vi "Process.vi"(8 "error in":errorcluster, 11 "SMO.Example":refnum<class "SMO.TopLevel.lvclass">) -> (0 "error out":errorcluster, 3 "SMO.Example out":refnum<class "SMO.TopLevel.lvclass">)   [LabVIEW 2013, in "SMO.TopLevel.lvclass"]
doc: "---------------------------------------------------------------\nJKI State Machine Objects™\nhttp://jki.net/state-machine-objects/\nCopyright (C) 2005-2015, JKI <info@jki.net>\nALL RIGHTS RESERVED"
uses:
  SMO.TopLevel.lvclass
  src/SMO/Typedefs/Parent Call--Enum.ctl
  src/SMO/SMO.lvclass
panel:
  # "For instructions on how to use the JKI State Machine Objects, examples and video tutorials, visit:\nhttp://jki.net/state-machine-objects/\n\nJKI State Machine Objects™\nhttp://jki.net/state-machine-objects/\nCopyright (C) 2005-2015, JKI <info@jki.net>\nALL RIGHTS RESERVED"
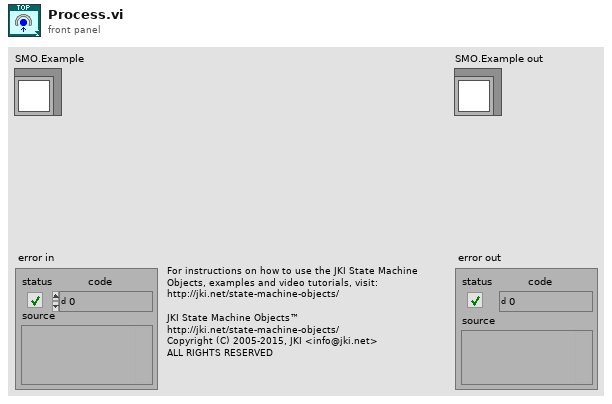
[diagram p1: front panel]
types:
  T1 = typedef "SMO.lvclass/Parent Call--Enum.ctl" = enum16{"Allows parent to run", "Does not request parent to run"}
  T2 = enum32{"invalid app kind", "Development System", "Run Time System", "Student Edition", "Embedded LabVIEW", "Evaluation", "Custom"}
  T3 = enum32{"Invalid", "Standard", "Closed", "Hidden", "Minimized", "Maximized"}
  T4 = cluster{"Core":cluster{"Current VI Reference":refnum<vi>, "Close Panel on Exit?":bool, "error":errorcluster}, "Self Ref":refnum<class "SMO.TopLevel.lvclass">, "Your string data":string, "Pump State":bool, "Valve 1 State":bool, "Flow 1 Actual":dbl, "Flow 2 Actual":dbl, "Flow 1 Target":dbl, "Flow 2 Target":dbl}
  T5 = cluster{"Current VI Reference":refnum<vi>, "Close Panel on Exit?":bool, "error":errorcluster}
  T6 = typedef "SMO.lvclass/Protected Events.ctl" = cluster{"StopProcesses":refnum<user-event>, "AbortProcesses":refnum<user-event>, "Config Changed":refnum<user-event>}
  T7 = typedef "SMO.TopLevel.lvclass/ProtectedEvents--Cluster.ctl" = cluster{"API_Template":refnum<user-event>, "PumpState":refnum<user-event>, "Valve State":refnum<user-event>}
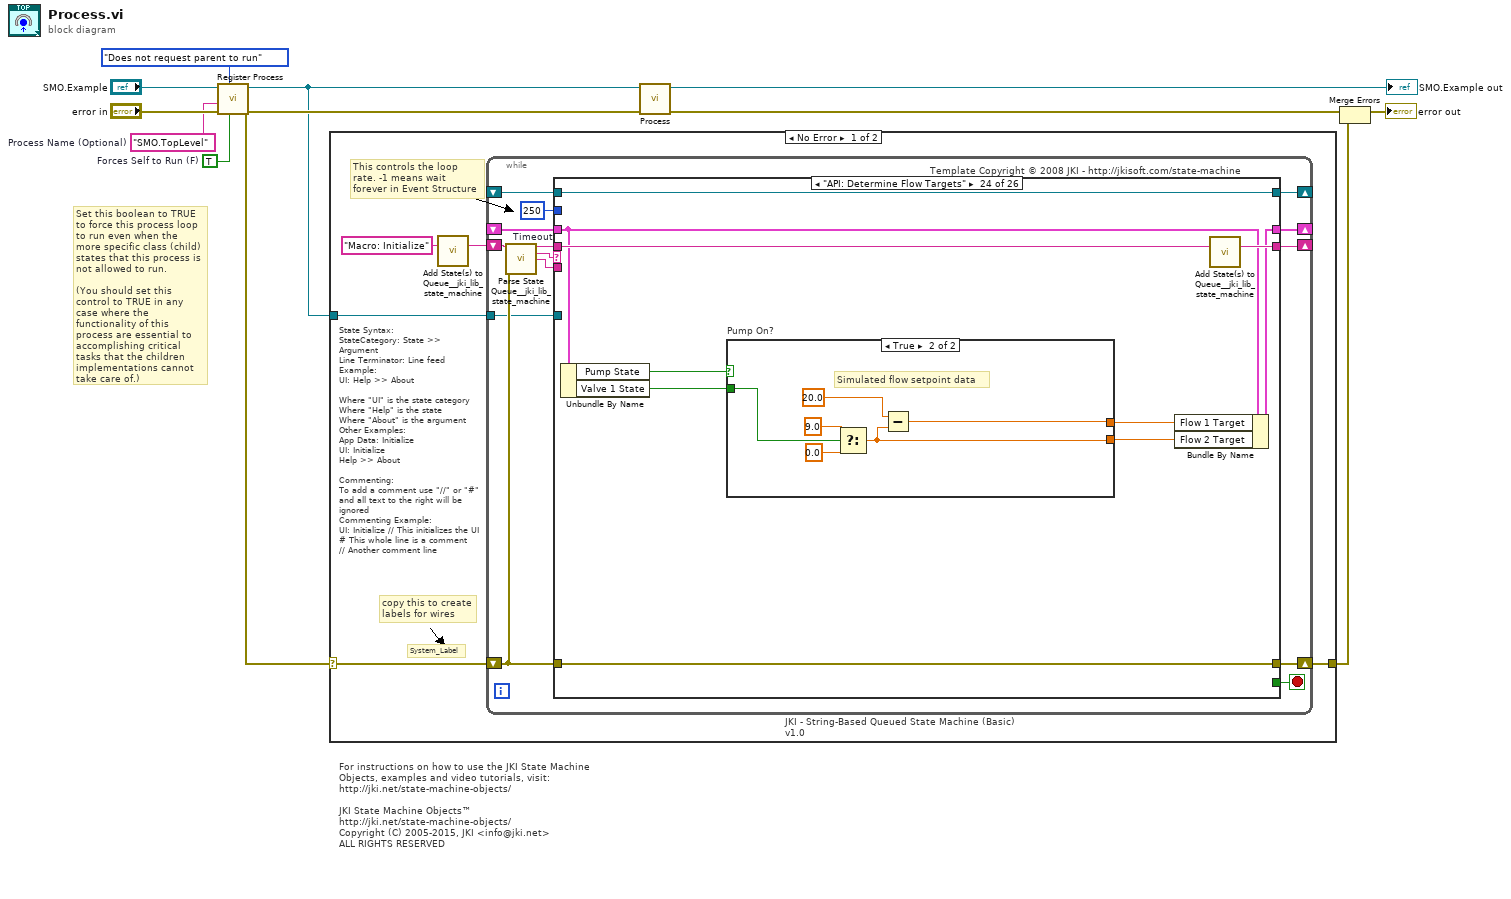
[diagram p0: block diagram]
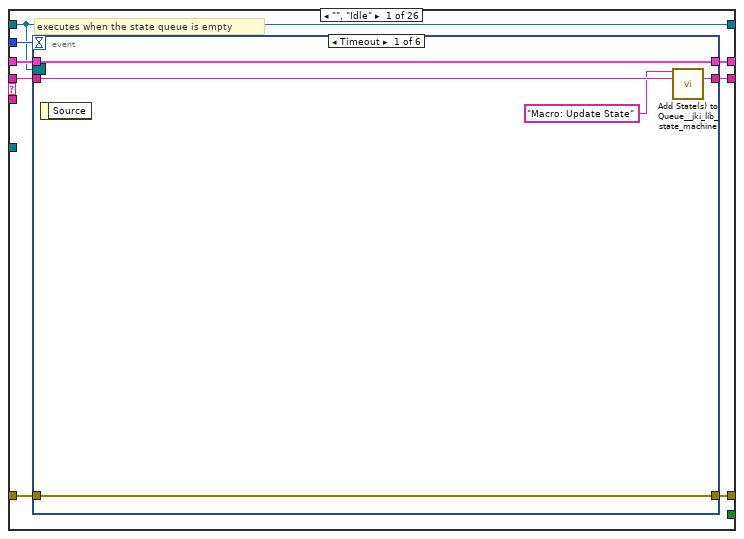
[diagram p2: hidden frame]
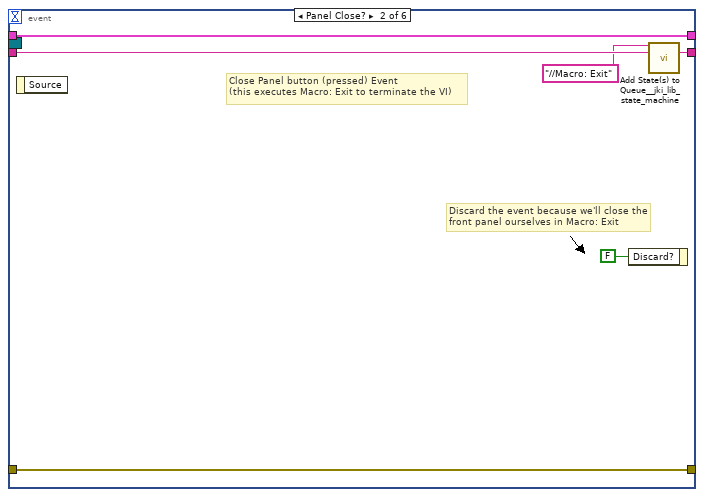
[diagram p3: hidden frame]
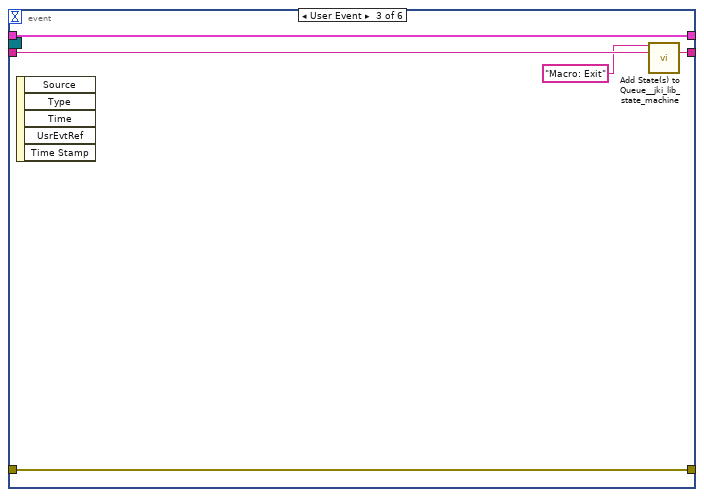
[diagram p4: hidden frame]
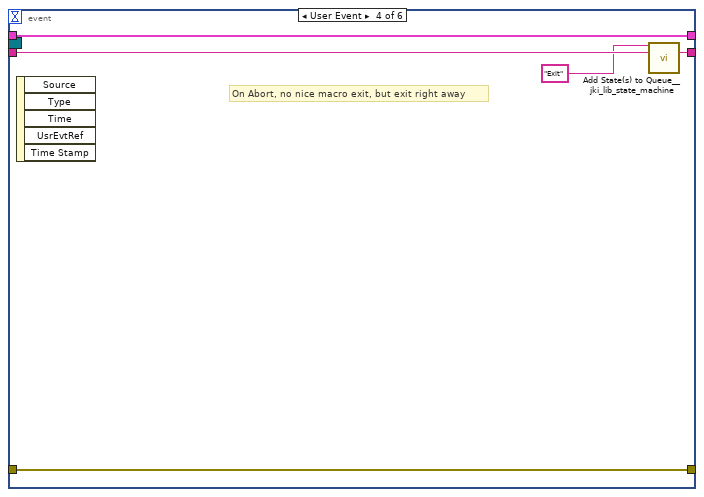
[diagram p5: hidden frame]
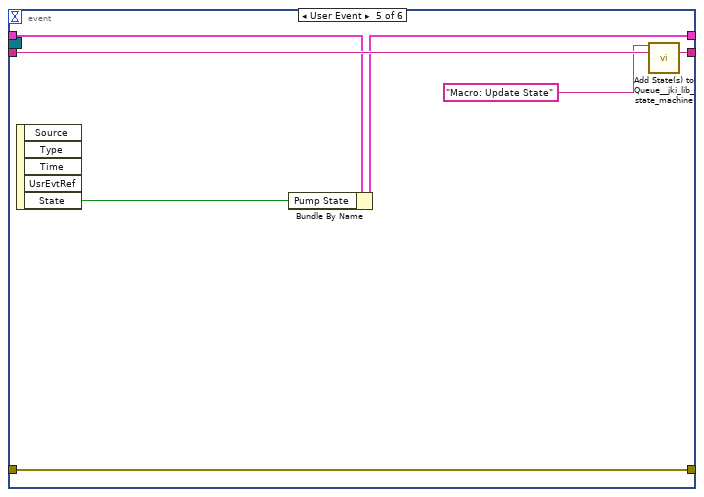
[diagram p6: hidden frame]
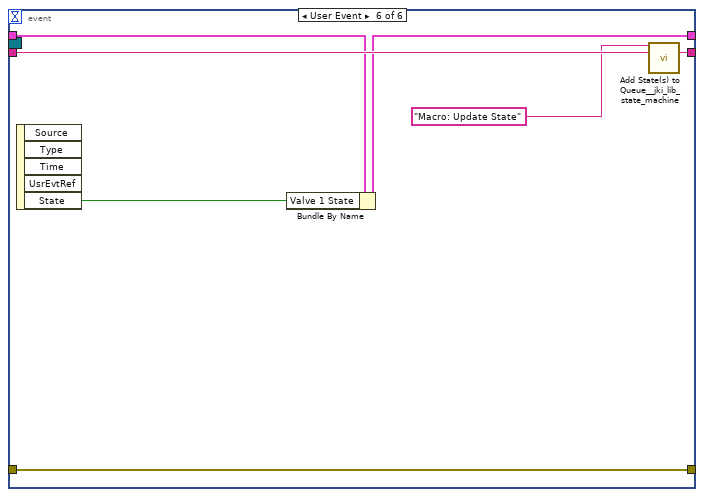
[diagram p7: hidden frame]
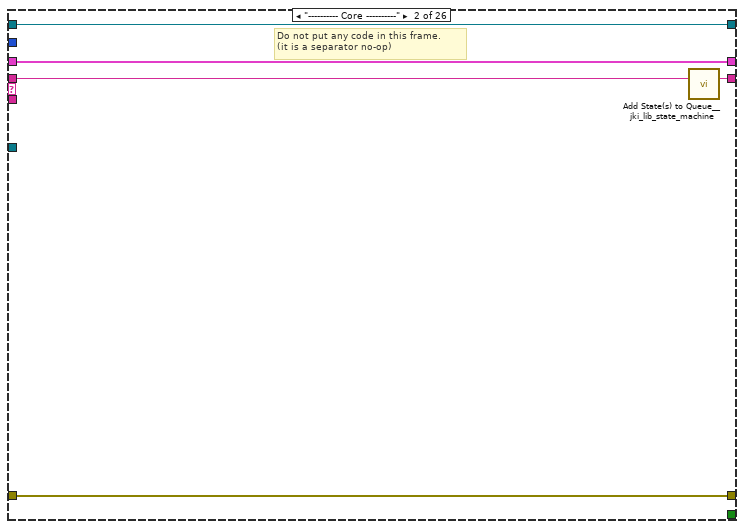
[diagram p8: hidden frame]
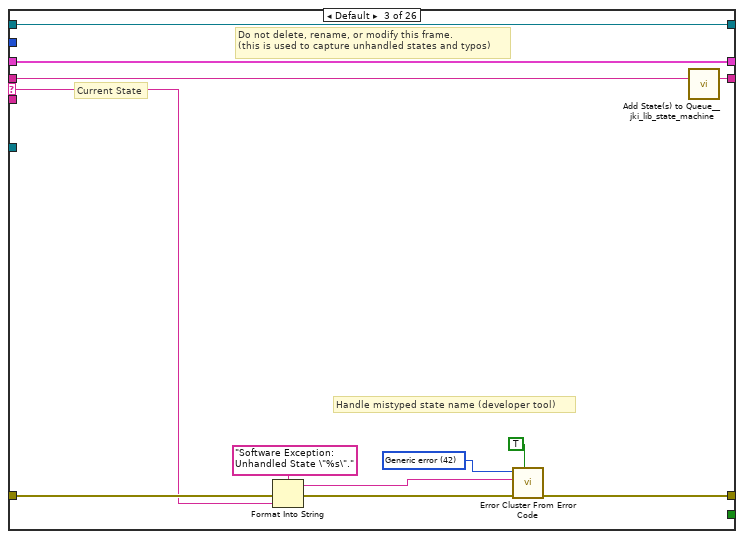
[diagram p9: hidden frame]
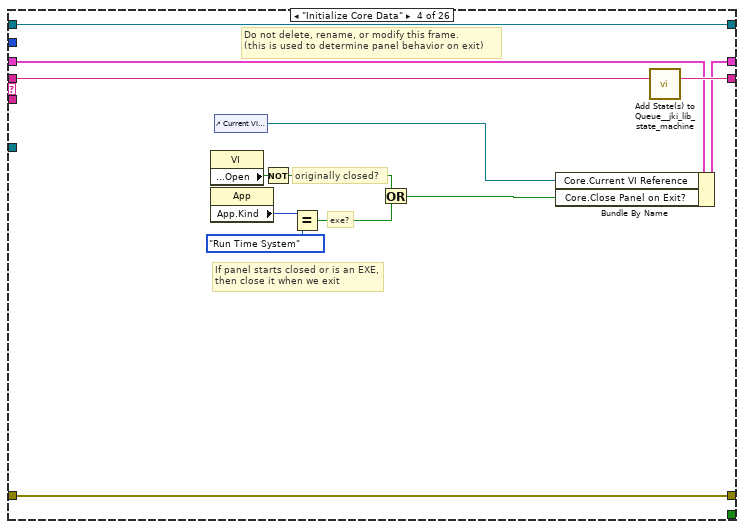
[diagram p10: hidden frame]
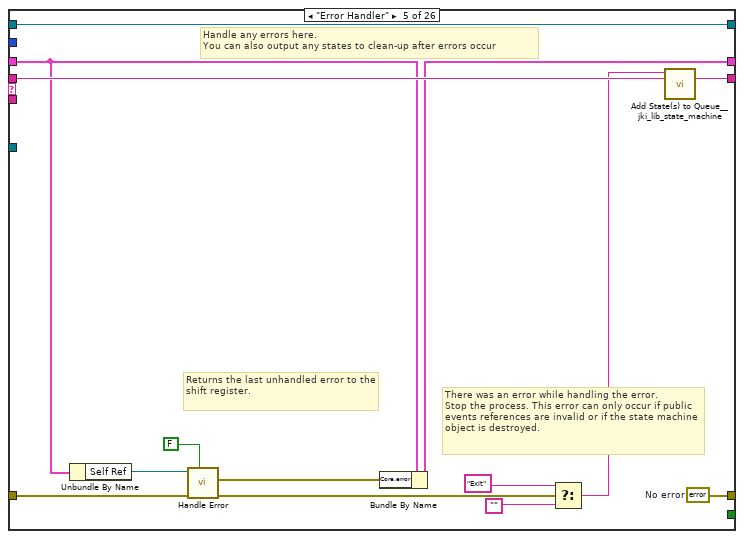
[diagram p11: hidden frame]
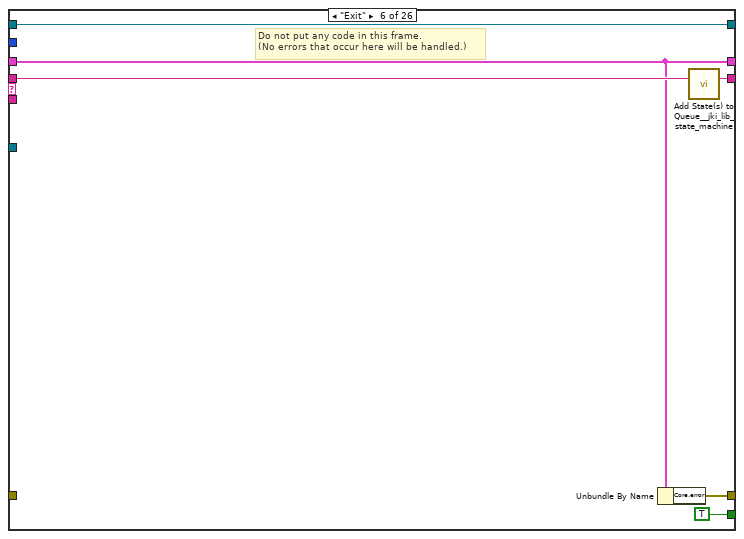
[diagram p12: hidden frame]
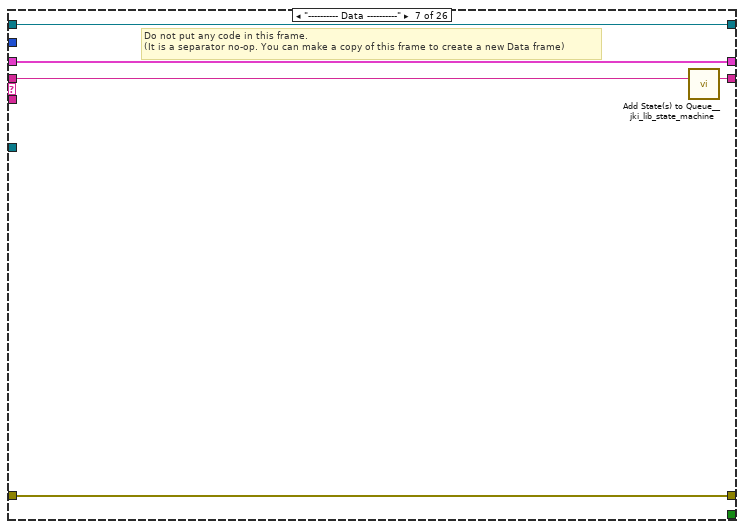
[diagram p13: hidden frame]
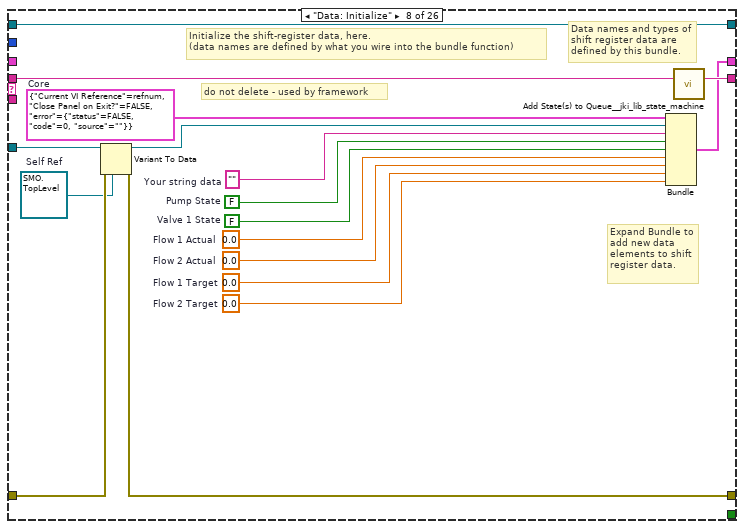
[diagram p14: hidden frame]
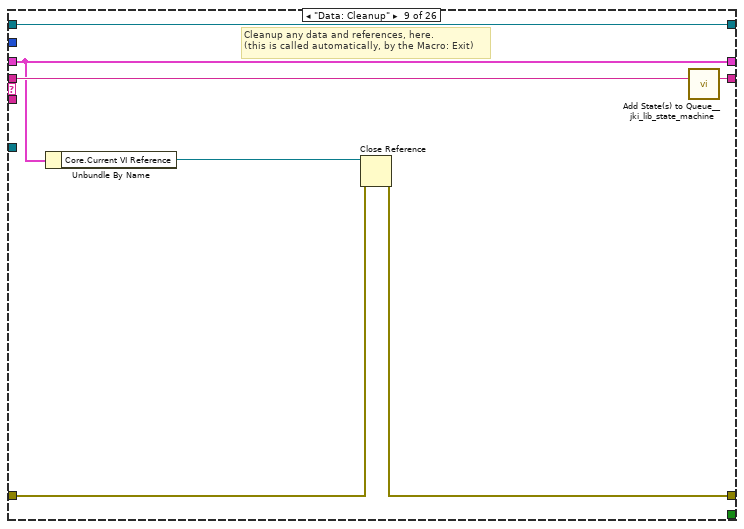
[diagram p15: hidden frame]
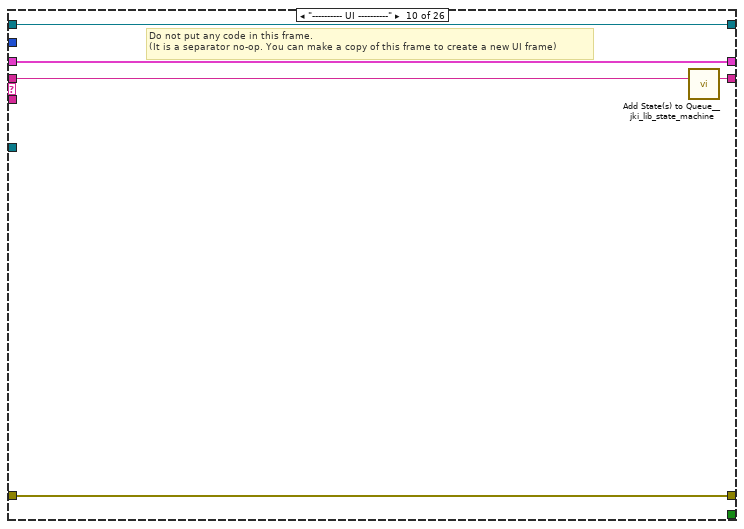
[diagram p16: hidden frame]
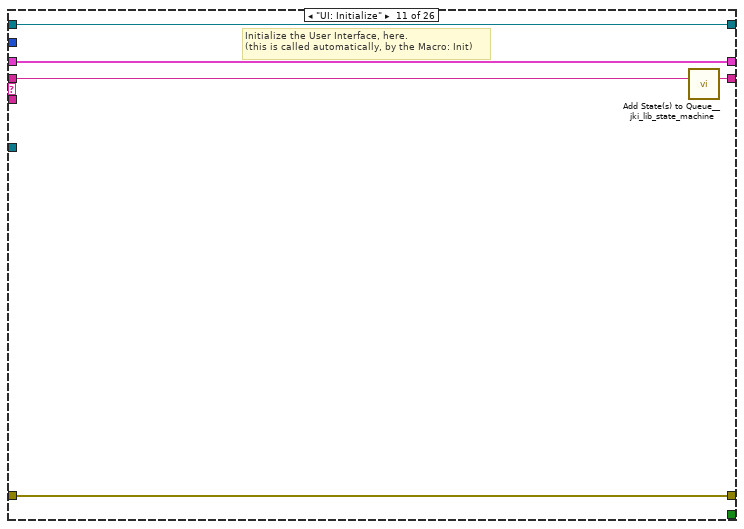
[diagram p17: hidden frame]
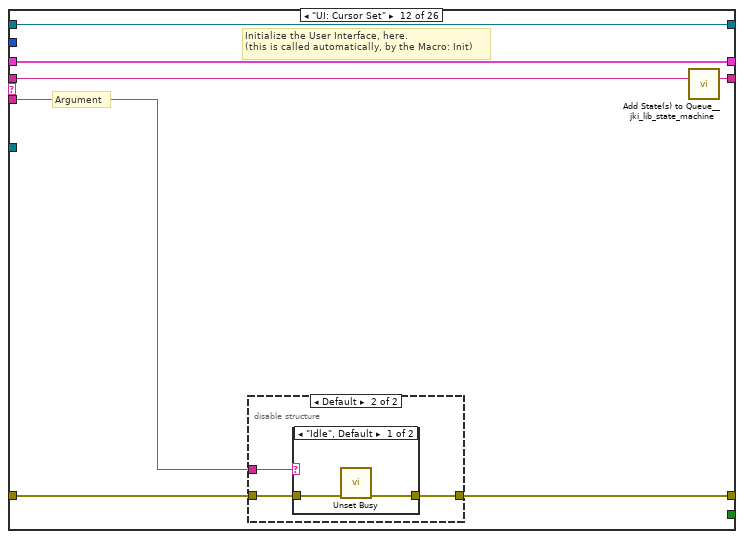
[diagram p18: hidden frame]
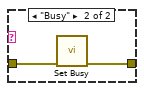
[diagram p20: hidden frame]
diagram:
  w1 = TRUE  # Forces Self to Run (F)
  w2 = "SMO.TopLevel"  # Process Name (Optional)
  # "Set this boolean to TRUE to force this process loop to run even when the more specific class (child) states that this process is not allowed to run.\n\n(You should set this control to TRUE in any case where the functionality of this process are essential to accomplishing critical tasks that the children implementations cannot take care of.)"
  # "For instructions on how to use the JKI State Machine Objects, examples and video tutorials, visit:\nhttp://jki.net/state-machine-objects/\n\nJKI State Machine Objects™\nhttp://jki.net/state-machine-objects/\nCopyright (C) 2005-2015, JKI <info@jki.net>\nALL RIGHTS RESERVED"
  n1 = call "Register Process.vi"("Forces Self to Run (F)"=w1, "Parent Call"=Parent_Call--Enum."Does not request parent to run", "error in (no error)"="error in", "Process Name (optional)"=w2, "SMO"="SMO.Example") -> ("error out"=w8:errorcluster, "SMO out"=w7:refnum<class "SMO.TopLevel.lvclass">)  [unwired: 5 in]
  n2 = case shown="No Error" w8 {
    selector: w8 -> [w13 w347]
    tunnel: w7 -> [w14 _]
    tunnel: [w12 w347] -> w4
    frame No Error {
      # "State Syntax:\nStateCategory: State >> Argument\nLine Terminator: Line feed\nExample:\nUI: Help >> About\n\nWhere \"UI\" is the state category\nWhere \"Help\" is the state\nWhere \"About\" is the argument\nOther Examples:\nApp Data: Initialize\nUI: Initialize\nHelp >> About\n\nCommenting:\nTo add a comment use \"//\" or \"#\" and all text to the right will be ignored\nCommenting Example:\nUI: Initialize // This initializes the UI\n# This whole line is a comment\n// Another comment line"
      # "copy this to create labels for wires"
      # "This controls the loop rate. -1 means wait forever in Event Structure"
      # "System_Label"
      n3 = call <vilib>:"Add State(s) to Queue__jki_lib_state_machine.vi"("State(s) in (\"\")"="Macro: Initialize") -> ("States Out"=w16:string)  [unwired: 14 in]
      n4 = while "JKI - String-Based Queued State Machine (Basic) v1.0" {
        shift-right: [w23] -> _
        shift-left: _ -> [w22]
        shift-right: [w26] -> w12
        shift-left: w13 -> [w20]
        shift-right: [w25] -> _
        shift-left: w16 -> [w27]
        tunnel: w14 -> [w19]
        shift-right: [w18] -> _
        shift-left: _ -> [w17]
        stop <- w24 stop-if-true
        w21 = 250  # Timeout
        # "Template Copyright © 2008 JKI - http://jkisoft.com/state-machine"
        n5 = call <vilib>:"Parse State Queue__jki_lib_state_machine.vi"("State Queue"=w27, "Error In (no error)"=w20) -> ("Remaining States"=w29:string, "Current State"=w30:string, "Arguments"=w28:string)  [unwired: 11 in]
        n6 = case shown="\"API: Determine Flow Targets\"" w30 {
          selector: w30 -> [_ _ w80 _ _ _ _ _ _ _ _ _ _ _ _ _ _ _ _ _ _ _ _ _ _ _]
          tunnel: w29 -> [w38 w78 w84 w103 w117 w123 w128 w145 w152 w157 w162 w169 w185 w217 w223 w232 w246 w251 w262 w267 w280 w286 w291 w301 w337 w346]
          tunnel: w28 -> [_ _ _ _ _ _ _ _ _ _ _ w163 w178 _ _ _ _ _ _ _ _ _ _ _ _ _]
          tunnel: w22 -> [w36 w75 w82 w94 w108 w119 w125 _ w147 w154 w160 w167 w183 w214 w220 w228 w237 w248 w259 w264 w278 w284 w289 w295 w333 w343]
          tunnel: [w35 w76 w86 w100 w105 w118 w126 w140 w148 w155 w159 w164 w179 w215 w221 w230 w244 w249 w253 w265 w268 w282 w287 w296 w334 w340] -> w26
          tunnel: w20 -> [w34 w76 w85 w100 w109 _ w126 w141 w149 w155 w159 w165 w180 w215 w221 w230 w244 w249 w254 w265 w269 w282 w287 w296 w334 w341]
          tunnel: [w37 w77 w83 w102 w116 w122 w127 w144 w151 w156 w161 w168 w184 w216 w222 w231 w245 w250 w261 w266 w279 w285 w290 w300 w336 w345] -> w25
          tunnel: [_ _ _ _ _ TRUE _ _ _ _ _ _ _ _ _ _ _ _ _ _ _ _ _ _ _ _] -> w24
          tunnel: [w33 w75 w82 w101 w107 w119 w125 w143 w147 w154 w160 w167 w183 w214 w220 w228 w237 w248 w259 w264 w278 w284 w289 w294 w332 w343] -> w23
          tunnel: w21 -> [w32 _ _ _ _ _ _ _ _ _ _ _ _ _ _ _ _ _ _ _ _ _ _ _ _ _]
          tunnel: w19 -> [_ _ _ _ _ _ _ w138 _ _ _ _ _ _ _ _ _ _ _ _ _ _ _ _ _ _]
          tunnel: [w31 w74 w79 w91 w115 w120 w124 w136 w146 w153 w158 w166 w182 w213 w219 w229 w238 w247 w260 w263 w274 w283 w288 w299 w335 w344] -> w18
          tunnel: w17 -> [w31 w74 w79 w91 w115 w120 w124 w136 w146 w153 w158 w166 w182 w213 w219 w229 w238 w247 w260 w263 _ w283 w288 w299 w335 w344]
          frame "", "Idle" {
            # "executes when the state queue is empty"
            n7 = event shown="[0] Timeout" {
              selector: w31 -> [_ _ _ _ _ _]
              dyn-events: _ -> [_ _ _ _ _ _]
              timeout: w32 -> [_ _ _ _ _ _]
              tunnel: w38 -> [w43 w49 w54 w59 w66 w73]
              tunnel: [w42 w48 w53 w58 w65 w72] -> w37
              tunnel: w36 -> [w40 w46 w51 w56 w63 w70]
              tunnel: [w41 w47 w52 w57 w64 w71] -> w35
              tunnel: w34 -> [w41 w47 w52 w57 w64 w71]
              tunnel: [w40 w46 w51 w56 w62 w69] -> w33
              event Timeout {
                n8 = event-data() -> ()  [unwired: 1 in, 1 out]
                n9 = call <vilib>:"Add State(s) to Queue__jki_lib_state_machine.vi"("State(s) in Front (\"\")"="Macro: Update State", "State(s) in (\"\")"=w43) -> ("States Out"=w42:string)  [unwired: 13 in]
              }
              event Panel Close? {
                # "Discard the event because we'll close the front panel ourselves in Macro: Exit"
                # "Close Panel button (pressed) Event\n(this executes Macro: Exit to terminate the VI)"
                n10 = event-data() -> ()  [unwired: 1 in, 1 out]
                n11 = event-data("Discard?"=FALSE) -> ()  [unwired: 1 in, 1 out]
                n12 = call <vilib>:"Add State(s) to Queue__jki_lib_state_machine.vi"("State(s) in Front (\"\")"="//Macro: Exit", "State(s) in (\"\")"=w49) -> ("States Out"=w48:string)  [unwired: 13 in]
              }
              event User Event {
                n13 = event-data() -> ()  [unwired: 1 in, 5 out]
                n14 = call <vilib>:"Add State(s) to Queue__jki_lib_state_machine.vi"("State(s) in Front (\"\")"="Macro: Exit", "State(s) in (\"\")"=w54) -> ("States Out"=w53:string)  [unwired: 13 in]
              }
              event User Event {
                # "On Abort, no nice macro exit, but exit right away"
                n15 = event-data() -> ()  [unwired: 1 in, 5 out]
                n16 = call <vilib>:"Add State(s) to Queue__jki_lib_state_machine.vi"("State(s) in Front (\"\")"="Exit", "State(s) in (\"\")"=w59) -> ("States Out"=w58:string)  [unwired: 13 in]
              }
              event User Event {
                n17 = event-data() -> ("State"=w60:bool)  [unwired: 1 in, 4 out]
                n18 = Bundle By Name(cluster=w63, "Pump State"=w60) -> (w62:T4)
                n19 = call <vilib>:"Add State(s) to Queue__jki_lib_state_machine.vi"("State(s) in Front (\"\")"="Macro: Update State", "State(s) in (\"\")"=w66) -> ("States Out"=w65:string)  [unwired: 13 in]
              }
              event User Event {
                n20 = event-data() -> ("State"=w67:bool)  [unwired: 1 in, 4 out]
                n21 = Bundle By Name(cluster=w70, "Valve 1 State"=w67) -> (w69:T4)
                n22 = call <vilib>:"Add State(s) to Queue__jki_lib_state_machine.vi"("State(s) in Front (\"\")"="Macro: Update State", "State(s) in (\"\")"=w73) -> ("States Out"=w72:string)  [unwired: 13 in]
              }
            }
          }
          frame "---------- Core ----------" {
            # "Do not put any code in this frame.\n(it is a separator no-op)"
            n23 = call <vilib>:"Add State(s) to Queue__jki_lib_state_machine.vi"("State(s) in (\"\")"=w78) -> ("States Out"=w77:string)  [unwired: 14 in]
          }
          frame Default {
            w89 = 42 items=["No error", "Argument error", "Memory is full", "Out of zone", "End of file", "File already open", "Generic file I/O error", "File not found", "File permission error", "Disk is full", "Duplicate path", "Too many files open", "System feature not enabled", "Resource file not found", "Cannot add resource", "Resource not found", "Image not found", "Image memory error", "Pen does not exist", "Config type invalid", "Config token not found", "Config parse error", "Config memory error", "Bad external code format", "Bad external code offset", "External code not present", "Null window", "Destroy window error", "Null menu", "Print aborted", "Bad print record", "Print driver error", "Windows error during printing", "Memory error during printing", "Print dialog error", "Generic print error", "Invalid device refnum", "Device not found", "Device parameter error", "Device unit error", "Cannot open device", "Device call aborted", "Generic error", "Cancelled by user", "Object ID too low", "Object ID too high", "Object not in heap", "Unknown heap", "Unknown object (invalid DefProc)", "Unknown object (DefProc not in table)", "Message out of range", "Invalid (null) method", "Unknown message", "Manager call not supported", "Bad address", "Network operation in progress", "Network operation timed out", "Connection is busy", "Network attribute not supported", "Network error", "Address in use", "System out of memory", "Connection aborted", "Connection refused", "Not connected", "Already connected", "Connection closed", "Initialization error (interapplication manager)", "Bad occurrence", "Wait on unbound occurrence handler", "Occurrence queue overflow", "Datalog type conflict", "Unused", "Unrecognized type (interapplication manager)", "Memory corrupt", "Failed to make temporary DLL", "Old CIN version", "Drag socket not found", "Failed to load drop-object", "Failed to register OLE object", "Failed to release OLE object", "Format specifier type mismatch", "Unknown format specifier", "Too few format specifiers", "Too many format specifiers", "Scan failed", "Newer CIN version", "Error converting to variant", "Runtime menu error", "Password tampered", "Variant attribute not found", "Incompatible variant data type", "Event data is not available", "Event Store is not present", "Occurrence is not found", "Event Queue is not created", "Event info is not available", "Refnum passed is NULL", "Error retrieving Class GUID", "Error retrieving CoClass GUID", "Error retrieving TypeLib GUID.", "Bad built application magic bytes.", "Specific driver is different from the specific driver associated with the Logical Name.", "There is no session opened to the class driver.", "Max Error", "MAX - Error with config objects", "MAX - Error loading configuration", "MAX - Group not supported"]
            # "Current State"
            # "Do not delete, rename, or modify this frame.\n(this is used to capture unhandled states and typos)"
            # "Handle mistyped state name (developer tool)"
            n24 = Format Into String(format string="Software Exception: Unhandled State \"%s\"." ("message"), error in=w85, w80) -> (resulting string=w88:string, error out=w87:errorcluster)  [unwired: 1 in]
            n25 = call <vilib>:"Error Cluster From Error Code.vi"("show call chain? (False)"=TRUE, "error in (no error)"=w87, "error message (\"\")"=w88, "error code (0)"=w89) -> ("error out"=w86:errorcluster)  [unwired: 5 in]
            n26 = call <vilib>:"Add State(s) to Queue__jki_lib_state_machine.vi"("State(s) in (\"\")"=w84) -> ("States Out"=w83:string)  [unwired: 14 in]
          }
          frame "Initialize Core Data" {
            # "Do not delete, rename, or modify this frame.\n(this is used to determine panel behavior on exit)"
            # "originally closed?"
            # "exe?"
            # "If panel starts closed or is an EXE, then close it when we exit"
            n27 = property class="VI"() -> ("Front Panel.Open"=w99:bool)  [unwired: 2 in, 2 out]
            n28 = property class="App"() -> ("App.Kind"=w98:T2)  [unwired: 2 in, 2 out]
            n29 = control-ref of="Current VI Reference"() -> (w92:refnum<vi>)
            n30 = Not(x=w99) -> (.not. x?=w96:bool)
            n31 = Equal?(x=w98, y=T2."Run Time System" ("Application:Kind")) -> (x = y?=w95:bool)
            n32 = Or(x=w96, y=w95) -> (x .or. y?=w93:bool)
            n33 = Bundle By Name(cluster=w94, "Core.Current VI Reference"=w92, "Core.Close Panel on Exit?"=w93) -> (w101:T4)
            n34 = call <vilib>:"Add State(s) to Queue__jki_lib_state_machine.vi"("State(s) in (\"\")"=w103) -> ("States Out"=w102:string)  [unwired: 14 in]
          }
          frame "Error Handler" {
            w105 = errorcluster {"status"=FALSE, "code"=0, "source"=""}  # No error
            # "Returns the last unhandled error to the shift register."
            # "There was an error while handling the error.\nStop the process. This error can only occur if public events references are invalid or if the state machine object is destroyed."
            # "Handle any errors here.\nYou can also output any states to clean-up after errors occur"
            n35 = Unbundle By Name(w108) -> ("Self Ref"=w110:refnum<class "SMO.TopLevel.lvclass">)
            n36 = call-dynamic "Handle Error.vi"("Stop on Unhandled Error (T)"=FALSE, "error in"=w109, "SMO"=w110) -> ("handling error"=w112:errorcluster, "Unhandled error"=w111:errorcluster)  [unwired: 6 in, 1 out]
            n37 = Bundle By Name(cluster=w108, "Core.error"=w111) -> (w107:T4)
            n38 = Select(t="Exit", s=w112, f="") -> (s? t:f=w106:string)
            n39 = call <vilib>:"Add State(s) to Queue__jki_lib_state_machine.vi"("State(s) in Front (\"\")"=w106, "State(s) in (\"\")"=w117) -> ("States Out"=w116:string)  [unwired: 13 in]
          }
          frame "Exit" {
            # "Do not put any code in this frame.\n(No errors that occur here will be handled.)"
            n40 = Unbundle By Name(w119) -> ("Core.error"=w118:errorcluster)
            n41 = call <vilib>:"Add State(s) to Queue__jki_lib_state_machine.vi"("State(s) in (\"\")"=w123) -> ("States Out"=w122:string)  [unwired: 14 in]
          }
          frame "---------- Data ----------" {
            # "Do not put any code in this frame.\n(It is a separator no-op. You can make a copy of this frame to create a new Data frame)"
            n42 = call <vilib>:"Add State(s) to Queue__jki_lib_state_machine.vi"("State(s) in (\"\")"=w128) -> ("States Out"=w127:string)  [unwired: 14 in]
          }
          frame "Data: Initialize" {
            w129 = T5 {"Current VI Reference"=refnum, "Close Panel on Exit?"=FALSE, "error"={"status"=FALSE, "code"=0, "source"=""}}  # Core
            w130 = 0.0  # Flow 2 Target
            w131 = 0.0  # Flow 1 Target
            w132 = 0.0  # Flow 2 Actual
            w133 = 0.0  # Flow 1 Actual
            w134 = FALSE  # Valve 1 State
            w135 = FALSE  # Pump State
            w139 = refnum<class "SMO.TopLevel.lvclass"> refnum  # Self Ref
            w142 = ""  # Your string data
            # "do not delete - used by framework"
            # "Expand Bundle to add new data elements to shift register data."
            # "Data names and types of shift register data are defined by this bundle."
            # "Initialize the shift-register data, here.\n(data names are defined by what you wire into the bundle function)"
            n43 = Variant To Data(error in=w141, type=w139, Variant=w138) -> (data=w137:refnum<class "SMO.TopLevel.lvclass">, error out=w140:errorcluster)
            n44 = Bundle("Core"=w129, "Self Ref"=w137, "Your string data"=w142, "Pump State"=w135, "Valve 1 State"=w134, "Flow 1 Actual"=w133, "Flow 2 Actual"=w132, "Flow 1 Target"=w131, "Flow 2 Target"=w130) -> (w143:T4)  [unwired: 1 in]
            n45 = call <vilib>:"Add State(s) to Queue__jki_lib_state_machine.vi"("State(s) in (\"\")"=w145) -> ("States Out"=w144:string)  [unwired: 14 in]
          }
          frame "Data: Cleanup" {
            # "Cleanup any data and references, here.\n(this is called automatically, by the Macro: Exit)"
            n46 = Unbundle By Name(w147) -> ("Core.Current VI Reference"=w150:refnum<vi>)
            n47 = Close Reference(reference=w150, error in (no error)=w149) -> (error out=w148:errorcluster)
            n48 = call <vilib>:"Add State(s) to Queue__jki_lib_state_machine.vi"("State(s) in (\"\")"=w152) -> ("States Out"=w151:string)  [unwired: 14 in]
          }
          frame "---------- UI ----------" {
            # "Do not put any code in this frame.\n(It is a separator no-op. You can make a copy of this frame to create a new UI frame)"
            n49 = call <vilib>:"Add State(s) to Queue__jki_lib_state_machine.vi"("State(s) in (\"\")"=w157) -> ("States Out"=w156:string)  [unwired: 14 in]
          }
          frame "UI: Initialize" {
            # "Initialize the User Interface, here.\n(this is called automatically, by the Macro: Init)"
            n50 = call <vilib>:"Add State(s) to Queue__jki_lib_state_machine.vi"("State(s) in (\"\")"=w162) -> ("States Out"=w161:string)  [unwired: 14 in]
          }
          frame "UI: Cursor Set" {
            # "Argument"
            # "Initialize the User Interface, here.\n(this is called automatically, by the Macro: Init)"
            n51 = disable-structure shown="Default" {
              disable-tunnel: w165 -> [w170 w173]
              disable-tunnel: [w170 w172] -> w164
              disable-tunnel: w163 -> [_ w171]
              frame condition #0 {
              }
              frame condition #1 (active) {
                n52 = case shown="\"Idle\", Default" w171 {
                  tunnel: w173 -> [w175 w177]
                  tunnel: [w174 w176] -> w172
                  frame "Idle", Default {
                    n53 = call <vilib>:"Unset Busy.vi"("error in (no error)"=w175) -> ("error out"=w174:errorcluster)  [unwired: 10 in]
                  }
                  frame "Busy" {
                    n54 = call <vilib>:"Set Busy.vi"("error in (no error)"=w177) -> ("error out"=w176:errorcluster)  [unwired: 9 in, 1 out]
                  }
                }
              }
            }
            n55 = call <vilib>:"Add State(s) to Queue__jki_lib_state_machine.vi"("State(s) in (\"\")"=w169) -> ("States Out"=w168:string)  [unwired: 14 in]
          }
          frame "UI: Front Panel State" {
            # "Argument"
            # "Set Front Panel Open or Closed\n(Usage: \"UI: Front Panel State >> Open|Close\")"
            n56 = Unbundle By Name(w183) -> ("Core.Current VI Reference"=w181:refnum<vi>)
            n57 = disable-structure shown="Default" {
              disable-tunnel: w180 -> [w189 w212]
              disable-tunnel: [w188 w212] -> w179
              disable-tunnel: w181 -> [w187 _]
              disable-tunnel: w178 -> [w186 _]
              frame condition #0 (active) {
                n58 = case shown="\"Open\"" w186 {
                  tunnel: w189 -> [w193 w206]
                  tunnel: [w195 w207] -> w188
                  tunnel: w187 -> [w194 w204]
                  frame "Open" {
                    # "Open FP if not open or invalid"
                    n59 = property class="VI"(reference=w194, error in=w193) -> (reference out=w191:refnum<vi>, error out=w192:errorcluster, "FP.State"=w190:T3)
                    n60 = case shown="Default" w190 {
                      tunnel: [w198 w201] -> w195
                      tunnel: w192 -> [w197 w201]
                      tunnel: w191 -> [w196 _]
                      frame Default {
                        n61 = invoke class="VI" method="FP.Open"(reference=w196, error in=w197, "Activate"=TRUE, "State"=T3."Standard") -> (error out=w198:errorcluster)  [unwired: 1 in, 4 out]
                      }
                      frame "Invalid", "Standard" {
                      }
                    }
                  }
                  frame "Close", Default {
                    # "Close FP is not Closed or Invalid"
                    n62 = property class="VI"(reference=w204, error in=w206) -> (reference out=w203:refnum<vi>, error out=w205:errorcluster, "FP.State"=w202:T3)
                    n63 = case shown="Default" w202 {
                      tunnel: [w208 w211] -> w207
                      tunnel: w205 -> [w208 w210]
                      tunnel: w203 -> [_ w209]
                      frame "Invalid", "Closed" {
                      }
                      frame Default {
                        n64 = invoke class="VI" method="FP.Close"(reference=w209, error in=w210) -> (error out=w211:errorcluster)  [unwired: 1 in, 2 out]
                      }
                    }
                  }
                }
              }
              frame condition #1 {
              }
            }
            n65 = call <vilib>:"Add State(s) to Queue__jki_lib_state_machine.vi"("State(s) in (\"\")"=w185) -> ("States Out"=w184:string)  [unwired: 14 in]
          }
          frame "---------- Macro ----------" {
            # "Do not put any code in this frame.\n(It is a separator no-op. You can make a copy of this frame to create a new Macro frame)"
            n66 = call <vilib>:"Add State(s) to Queue__jki_lib_state_machine.vi"("State(s) in (\"\")"=w217) -> ("States Out"=w216:string)  [unwired: 14 in]
          }
          frame "Macro: Update State" {
            n67 = call <vilib>:"Add State(s) to Queue__jki_lib_state_machine.vi"("State(s) in Front (\"\")"="API: Determine Flow Targets\nAPI: Determine Actual Flow\nAPI: Update State", "State(s) in (\"\")"=w223) -> ("States Out"=w222:string)  [unwired: 13 in]
          }
          frame "Macro: Initialize" {
            w226 = "UI: Initialize\n//UI: Front Panel State >> Open"  # UI: Initialize //UI: Front Panel State >> Open
            # "Initialization Macro\n(This is called once, when the VI starts)"
            n68 = call <vilib>:"Add State(s) to Queue__jki_lib_state_machine.vi"("State(s) in Front (\"\")"="Data: Initialize\nInitialize Core Data\nEvents: Register", "State(s) in (\"\")"="Process: Sync", "State(s) at Back (\"\")"=w226) -> ("States Out"=w225:string)  [unwired: 12 in]
            n69 = call <vilib>:"Add State(s) to Queue__jki_lib_state_machine.vi"("State(s) in Front (\"\")"=w225, "State(s) in (\"\")"=w232) -> ("States Out"=w231:string)  [unwired: 13 in]
          }
          frame "Macro: Exit" {
            # "Exit Macro\n(This is called once, when the VI exits)"
            n70 = Unbundle By Name(w237) -> ("Core.Close Panel on Exit?"=w243:bool)
            n71 = Select(t="//UI: Front Panel State >> Close", s=w243, f="") -> (s? t:f=w240:string)
            n72 = call <vilib>:"Add State(s) to Queue__jki_lib_state_machine.vi"("State(s) in Front (\"\")"="Data: Cleanup\nEvents: Unregister", "State(s) in (\"\")"="Process: Sync", "State(s) at Back (\"\")"="Exit") -> ("States Out"=w234:string)  [unwired: 12 in]
            n73 = call <vilib>:"Add State(s) to Queue__jki_lib_state_machine.vi"("State(s) in (\"\")"=w240, "State(s) at Back (\"\")"=w234) -> ("States Out"=w239:string)  [unwired: 13 in]
            n74 = call <vilib>:"Add State(s) to Queue__jki_lib_state_machine.vi"("State(s) in Front (\"\")"=w239, "State(s) in (\"\")"=w246) -> ("States Out"=w245:string)  [unwired: 13 in]
          }
          frame "---------- Process ----------" {
            # "Template Separator\n(You can make a copy of, or modify, this frame)"
            n75 = call <vilib>:"Add State(s) to Queue__jki_lib_state_machine.vi"("State(s) in (\"\")"=w251) -> ("States Out"=w250:string)  [unwired: 14 in]
          }
          frame "Process: Sync" {
            # "Template Separator\n(You can make a copy of, or modify, this frame)"
            n76 = Unbundle By Name(w259) -> ("Self Ref"=w255:refnum<class "SMO.TopLevel.lvclass">)
            n77 = call "WaitOnProcessSync.vi"("error in (no error)"=w254, "SMO"=w255) -> ("error out"=w253:errorcluster, "Don't run?"=w258:bool)  [unwired: 7 in, 1 out]
            n78 = Select(t="Data: Cleanup\nEvents: Unregister\nExit", s=w258, f="") -> (s? t:f=w252:string)
            n79 = call <vilib>:"Add State(s) to Queue__jki_lib_state_machine.vi"("State(s) in Front (\"\")"=w252, "State(s) in (\"\")"=w262) -> ("States Out"=w261:string)  [unwired: 13 in]
          }
          frame "---------- Events ----------" {
            # "Template Separator\n(You can make a copy of, or modify, this frame)"
            n80 = call <vilib>:"Add State(s) to Queue__jki_lib_state_machine.vi"("State(s) in (\"\")"=w267) -> ("States Out"=w266:string)  [unwired: 14 in]
          }
          frame "Events: Register" {
            # "Self Public Events"
            # "Base Class Protected Events"
            # "Your code here.\n(You can make a copy of, or modify, this frame)"
            n81 = Unbundle By Name(w278) -> ("Self Ref"=w277:refnum<class "SMO.TopLevel.lvclass">)
            n82 = call "GetProtectedEvents.vi"("SMO"=w277) -> ("error out"=w270:errorcluster, "SMO Protected Events"=w276:T6, "SMO out"=w275:refnum<class "SMO.TopLevel.lvclass">)  [unwired: 8 in]
            n83 = call "SMO.Example.GetProtectedEvents.vi"("SMO.Example"=w275) -> ("error out"=w271:errorcluster, "Protected Events"=w273:T7)  [unwired: 8 in, 1 out]
            n84 = register-events(w276, w273) -> (reference out=w274:refnum<event-registration>, error out=w272:errorcluster)  [unwired: 2 in]
            n85 = Merge Errors(w269, w272, w271, w270) -> (w268:errorcluster)
            n86 = call <vilib>:"Add State(s) to Queue__jki_lib_state_machine.vi"("State(s) in (\"\")"=w280) -> ("States Out"=w279:string)  [unwired: 14 in]
          }
          frame "Events: Unregister" {
            # "Your code here.\n(You can make a copy of, or modify, this frame)"
            n87 = Unregister For Events(event registration refnum=w283, error in=w282) -> (error out=w281:errorcluster)
            n88 = call <vilib>:"Clear Errors.vi"("error in (no error)"=w281) -> ()  [unwired: 6 in, 1 out]
            n89 = call <vilib>:"Add State(s) to Queue__jki_lib_state_machine.vi"("State(s) in (\"\")"=w286) -> ("States Out"=w285:string)  [unwired: 14 in]
          }
          frame "---------- API ----------" {
            n90 = call <vilib>:"Add State(s) to Queue__jki_lib_state_machine.vi"("State(s) in (\"\")"=w291) -> ("States Out"=w290:string)  [unwired: 14 in]
          }
          frame "API: Determine Flow Targets" {
            n91 = Unbundle By Name(w295) -> ("Pump State"=w298:bool, "Valve 1 State"=w297:bool)
            n92 = case "Pump On?" shown="True" w298 {
              tunnel: [w302 w306] -> w293
              tunnel: [w303 w305] -> w292
              tunnel: w297 -> [_ w309]
              frame False {
                w303 = 0.0  # Flow 2
                w302 = 0.0  # Flow 1
                # "If Pump is OFF, simulate no flow for either meter"
              }
              frame True {
                # "Simulated flow setpoint data"
                n93 = Select(t=9.0, s=w309, f=0.0) -> (s? t:f=w305:dbl)
                n94 = Subtract(x=20.0, y=w305) -> (x-y=w306:dbl)
              }
            }
            n95 = Bundle By Name(cluster=w295, "Flow 1 Target"=w293, "Flow 2 Target"=w292) -> (w294:T4)
            n96 = call <vilib>:"Add State(s) to Queue__jki_lib_state_machine.vi"("State(s) in (\"\")"=w301) -> ("States Out"=w300:string)  [unwired: 14 in]
          }
          frame "API: Determine Actual Flow" {
            # "asymptotically appraoch target value with each iteration"
            # "If target value for either is 0, don't add noise to that particular channel."
            # "Simulate flow rate data"
            n97 = Unbundle By Name(w333) -> ("Flow 1 Target"=w321:dbl, "Flow 1 Actual"=w322:dbl, "Flow 2 Target"=w310:dbl, "Flow 2 Actual"=w320:dbl)
            n98 = Equal To 0?(x=w321) -> (x = 0?=w314:bool)
            n99 = Equal To 0?(x=w310) -> (x = 0?=w318:bool)
            n100 = Random Number (0-1)() -> (number: 0 to 1=w315:dbl)
            n101 = Random Number (0-1)() -> (number: 0 to 1=w317:dbl)
            n102 = Select(t=0.0, s=w314, f=w315) -> (s? t:f=w312:dbl)
            n103 = Select(t=0.0, s=w318, f=w317) -> (s? t:f=w311:dbl)
            n104 = Subtract(x=w321, y=w322) -> (x-y=w331:dbl)
            n105 = Subtract(x=w310, y=w320) -> (x-y=w326:dbl)
            n106 = Divide(x=w331, y=4.0) -> (x/y=w329:dbl)
            n107 = Divide(x=w326, y=3.0) -> (x/y=w324:dbl)
            n108 = Add(x=w322, y=w329) -> (x+y=w328:dbl)
            n109 = Add(x=w320, y=w324) -> (x+y=w319:dbl)
            n110 = Add(x=w312, y=w328) -> (x+y=w327:dbl)
            n111 = Add(x=w319, y=w311) -> (x+y=w323:dbl)
            n112 = Bundle By Name(cluster=w333, "Flow 1 Actual"=w327, "Flow 2 Actual"=w323) -> (w332:T4)
            n113 = call <vilib>:"Add State(s) to Queue__jki_lib_state_machine.vi"("State(s) in (\"\")"=w337) -> ("States Out"=w336:string)  [unwired: 14 in]
          }
          frame "API: Update State" {
            n114 = Unbundle By Name(w343) -> ("Self Ref"=w342:refnum<class "SMO.TopLevel.lvclass">, "Flow 1 Actual"=w339:dbl, "Flow 2 Actual"=w338:dbl)
            n115 = call "SMO.Example.SetData.vi"("error in (no error)"=w341, "Flow 2"=w338, "Flow 1"=w339, "SMO.Example"=w342) -> ("error out"=w340:errorcluster)  [unwired: 6 in, 1 out]
            n116 = call <vilib>:"Add State(s) to Queue__jki_lib_state_machine.vi"("State(s) in (\"\")"=w346) -> ("States Out"=w345:string)  [unwired: 14 in]
          }
        }
      }
    }
    frame Error {
    }
  }
  n117 = call-parent "Process.vi"("error in"=w8, "SMO"=w7) -> ("error out"=w5:errorcluster, "SMO out"=→"SMO.Example out":refnum<class "SMO.TopLevel.lvclass">)  [unwired: 8 in]
  n118 = Merge Errors(w5, w4) -> (→"error out":errorcluster)
